vi "RX example.vi"() -> ()   [LabVIEW 2021]
uses:
  <vilib>/Analysis/2dsp.llb/Complex FFT.vi
  HackRF_Read_Complex.vi
  <vilib>/Analysis/NI_AALPro.lvlib
panel:
  out "Waveform Graph":dbl[](graph)
  in  "CarrierFreqHz":dbl(slide)=90658509.45494995 scale=86000000.0..110000000.0 scale format="%#_6p"
  in  "AMPEnable":bool
  in  "VGAGainDb":dbl=40.0 min=0.0 max=62.0 step=2.0
  in  "LNAGainDb":dbl=24.0 min=0.0 max=40.0 step=8.0
  in  "stop":bool
  in  "SampleFreqHz":dbl=4500000.0 format="%#_6p"
  in  "FilterBandwidthHz":dbl=3000000.0 format="%#_6p"
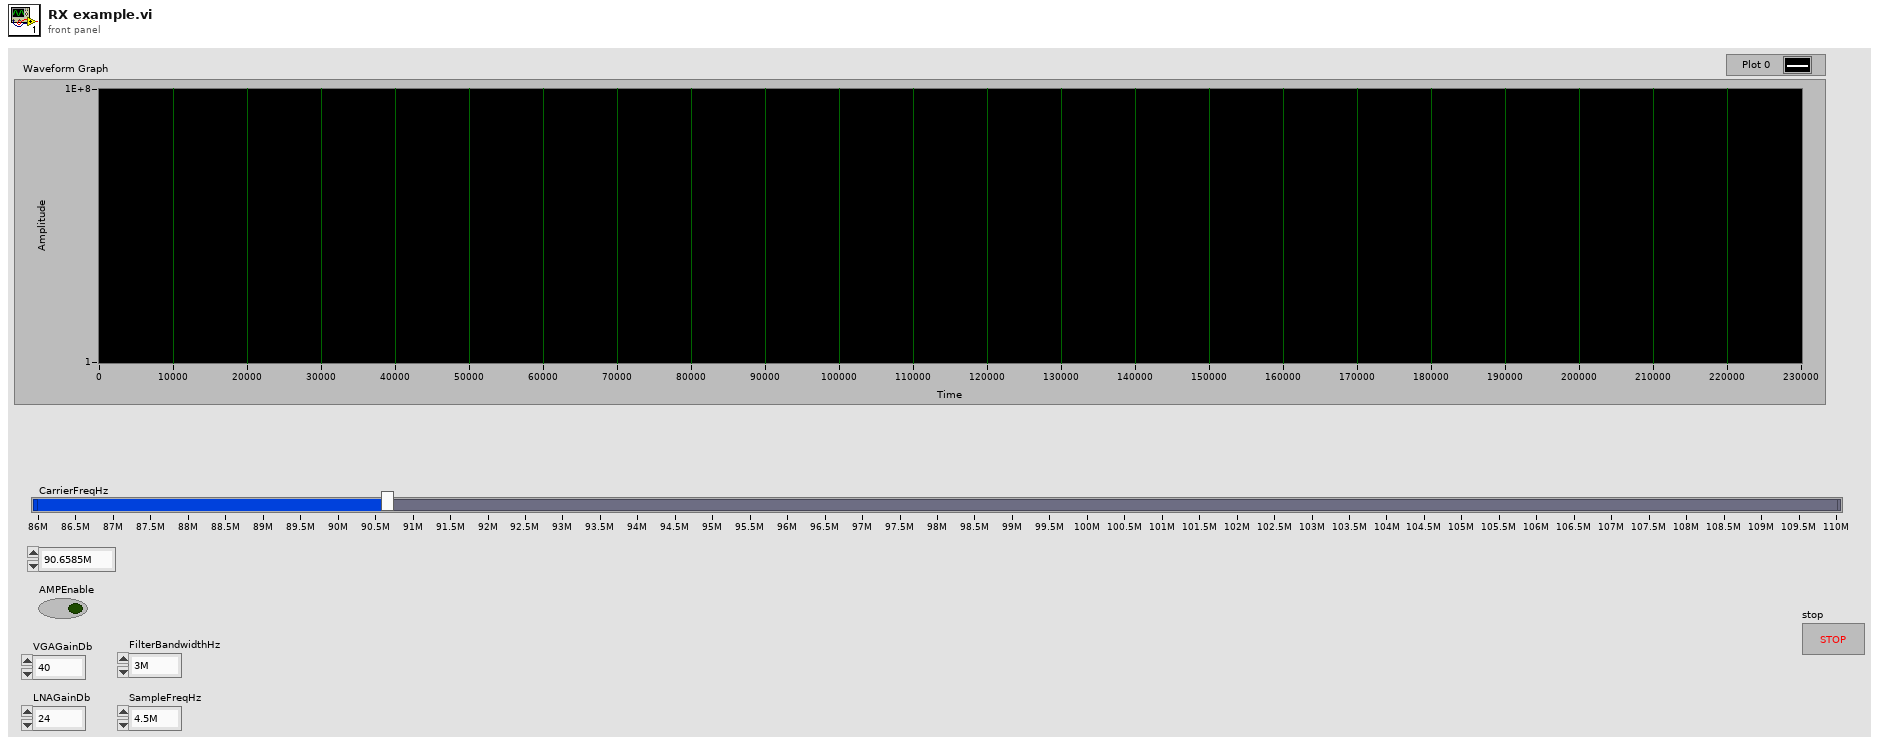
[diagram p1: front panel]
types:
  T1 = typedef "HackRF_Ref.ctl" = cluster{".net":refnum<k24>, "HackrfDeviceList":refnum<k24>[], "OpenDevice":refnum<k24>, "StartRX":refnum<k24>, "CarrierFreqHz":dbl, "SampleFreqHz":dbl, "FilterBandwidthHz":dbl, "AMPEnable":bool, "LNAGainDb":dbl, "VGAGainDb":dbl, "StartTx":refnum<k24>}
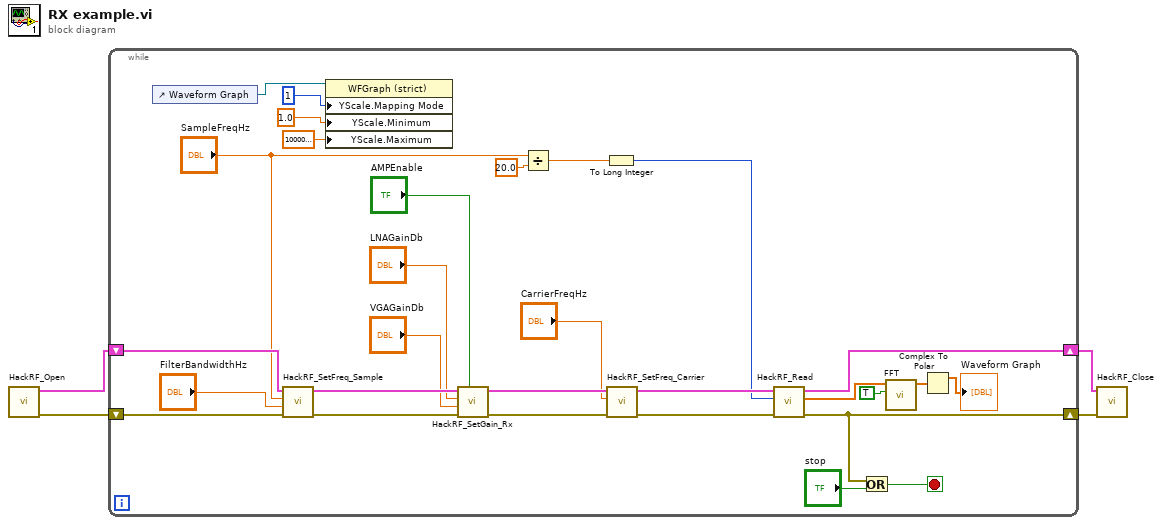
[diagram p0: block diagram]
diagram:
  n1 = call "HackRF_Open.vi"() -> ("error out"=w3:errorcluster, "Cluster"=w4:T1)  [unwired: 10 in]
  n2 = while {
    shift-right: [w17] -> w2
    shift-left: w4 -> [w33]
    shift-right: [w12] -> w1
    shift-left: w3 -> [w32]
    stop <- w10 stop-if-true
    n3 = control-ref of="Waveform Graph"() -> (w8:refnum<vi>)
    n4 = call "HackRF_SetFreq_Sample.vi"("error in (no error)"=w32, "FilterBandwidthHz"="FilterBandwidthHz", "SampleFreqHz"="SampleFreqHz", "HackRF in"=w33) -> ("error out"=w29:errorcluster, "HackRF out"=w30:T1)  [unwired: 6 in]
    n5 = property class="WFGraph (strict)"(reference=w8, "YScale.Mapping Mode"=u8 1 ("Y Scale.Mapping Mode"), "YScale.Minimum"=1.0 ("Y Scale.Range:Minimum"), "YScale.Maximum"=100000000.0 ("Y Scale.Range:Maximum")) -> ()  [unwired: 1 in, 2 out]
    n6 = call "HackRF_SetGain_Rx.vi"("AMPEnable"="AMPEnable", "error in (no error)"=w29, "VGAGainDb"="VGAGainDb", "LNAGainDb"="LNAGainDb", "HackRF in"=w30) -> ("error out"=w23:errorcluster, "HackRF out"=w26:T1)  [unwired: 5 in]
    n7 = Divide(x="SampleFreqHz", y=20.0) -> (x/y=w21:dbl)
    n8 = To Long Integer(number=w21) -> (32bit integer=w19:i32)
    n9 = call "HackRF_SetFreq_Carrier.vi"("error in (no error)"=w23, "CarrierFreqHz"="CarrierFreqHz", "HackRF_In"=w26) -> ("error out"=w18:errorcluster, "HackRF_Out"=w22:T1)  [unwired: 7 in]
    n10 = call-poly "HackRF_Read.vi"("error in (no error)"=w18, "count"=w19, "HackRF"=w22) -> ("error out"=w12:errorcluster, "Data"=w14:cdb[], "HackRF"=w17:T1)  [unwired: 6 in]
    n11 = Or(x=w12, y="stop") -> (x .or. y?=w10:bool)
    n12 = call-poly <vilib>:"FFT.vi"("shift?"=TRUE, "X"=w14) -> ("FFT {X}"=w13:cdb[])  [unwired: 8 in, 1 out]
    n13 = Complex To Polar(r * e^(i*theta)=w13) -> (r=→"Waveform Graph":dbl[])  [unwired: 1 out]
  }
  n14 = call "HackRF_Close.vi"("error in (no error)"=w1, "Cluster in"=w2) -> ()  [unwired: 8 in, 2 out]
